vi "Init Timer.vi"(8 "error in (no error)":errorcluster, 11 "AM Refs in in":T1) -> (0 "error out":errorcluster, 3 "AM Refs out":T1)   [LabVIEW 2020, in "Valve Control.lvlib"]
uses:
  Valve Control.lvlib
  AM Configuration.ctl
  support/Message Queue/Message Cluster.ctl
  support/Message Queue/Message Queue.lvlib
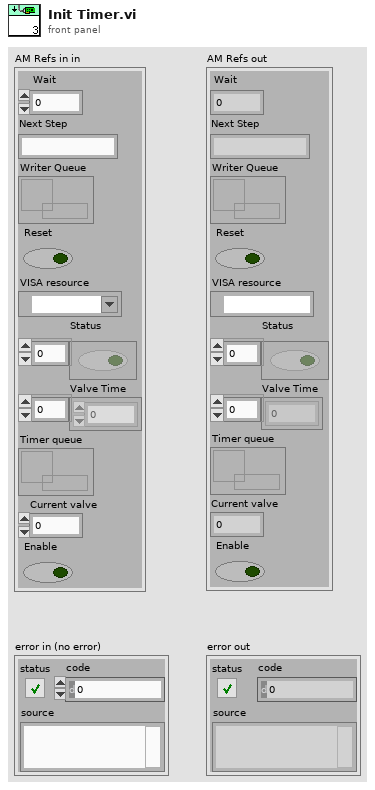
[diagram p1: front panel]
types:
  T1 = typedef "Valve Control.lvlib/AM Configuration.ctl" = cluster{"Wait":dbl, "Next Step":string, "Writer Queue":refnum<queue>, "Reset":bool, "VISA resource":refnum<visa-resource-name>, "Status":bool[], "Valve Time":dbl[], "Timer queue":refnum<queue>, "Current valve":i32, "Enable":bool}
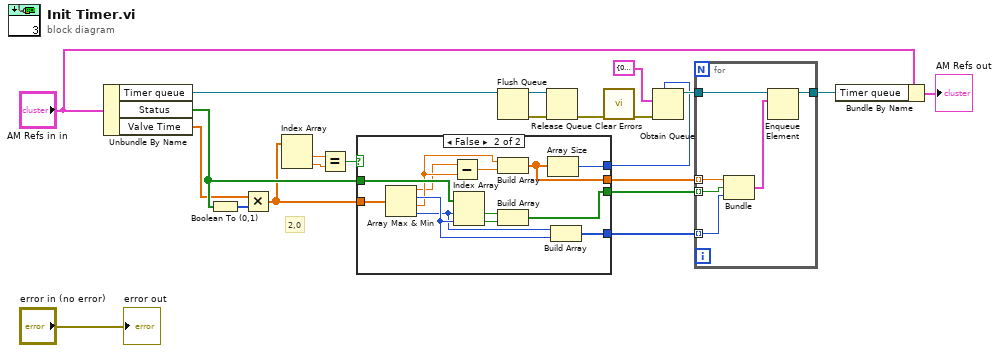
[diagram p0: block diagram]
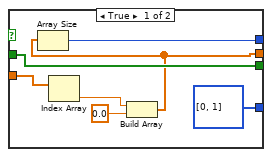
[diagram p2: hidden frame]
diagram:
  # "2,0"
  n1 = Unbundle By Name("AM Refs in in") -> ("Timer queue"=w17:refnum<queue>, "Status"=w21:bool[], "Valve Time"=w5:dbl[])
  n2 = Boolean To (0,1)(Boolean=w21) -> (0, 1=w22:i16[])
  n3 = Multiply(x=w5, y=w22) -> (x*y=w2:dbl[])
  n4 = Index Array(array=w2) -> (element #1=w4:dbl, element #2=w3:dbl)  [unwired: 2 in]
  n5 = Equal?(x=w4, y=w3) -> (x = y?=w1:bool)
  n6 = case shown="False" w1 {
    tunnel: w21 -> [w28 w42]
    tunnel: [i32[] [0, 1] ("appended array") w41] -> w19
    tunnel: [w28 w38] -> w18
    tunnel: [w23 w35] -> w14
    tunnel: [w29 w31] -> w7
    tunnel: w2 -> [w26 w30]
    frame True {
      n7 = Index Array(array=w26) -> (element=w25:dbl)  [unwired: 1 in]
      n8 = Build Array(w25, 0.0 ("element")) -> (w23:dbl[])
      n9 = Array Size(array=w23) -> (size(s)=w29:i32)
    }
    frame False {
      n10 = Array Max & Min(array=w30) -> (max value=w32:dbl, max index (indices)=w40:i32, min value=w33:dbl, min index (indices)=w39:i32)
      n11 = Subtract(x=w32, y=w33) -> (x-y=w34:dbl)
      n12 = Index Array(array=w42, index #1=w39, index #2=w40) -> (element #1=w36:bool, element #2=w37:bool)
      n13 = Build Array(w33, w34) -> (w35:dbl[])
      n14 = Build Array(w36, w37) -> (w38:bool[])
      n15 = Array Size(array=w35) -> (size(s)=w31:i32)
      n16 = Build Array(w39, w40) -> (w41:i32[])
    }
  }
  n17 = Flush Queue(queue=w17) -> (queue out=w9:refnum<queue>, error out=w10:errorcluster)  [unwired: 1 in, 1 out]
  n18 = Release Queue(queue=w9, error in (no error)=w10) -> (error out=w8:errorcluster)  [unwired: 1 in, 2 out]
  n19 = call <vilib>:"Clear Errors.vi"("error in (no error)"=w8) -> ("error out"=w12:errorcluster)  [unwired: 5 in, 1 out]
  n20 = Obtain Queue(max queue size (-1, unlimited)=w7, element data type=cluster{"Time":dbl, "Status":bool, "index":i32} {"Time"=0.0, "Status"=FALSE, "index"=0} ("output cluster"), error in (no error)=w12) -> (queue out=w11:refnum<queue>)  [unwired: 2 in, 2 out]
  n21 = for {
    tunnel: w11 -> [w47]
    tunnel: [w48] -> w16
    tunnel: w14 -> [w45] mode=indexing
    tunnel: w18 -> [w44] mode=indexing
    tunnel: w19 -> [w43] mode=indexing
    n22 = Bundle("element"=w45, "Status"=w44, w43) -> (w46:cluster{"element":dbl, "Status":bool, i32})  [unwired: 1 in]
    n23 = Enqueue Element(queue=w47, element=w46) -> (queue out=w48:refnum<queue>)  [unwired: 2 in, 2 out]
  }
  n24 = Bundle By Name(cluster="AM Refs in in", "Timer queue"=w16) -> (→"AM Refs out":T1)
  "error out" <- "error in (no error)"
